vi "Alarm Logical Channel.vi"(8 "error in (no error)":errorcluster, 9 "12 Logicals inputs state":T1[](array[typedef]) items=["Off", "On", "Ignore"], 10 "Alarm":u16(ring) items=["A", "B", "C", "D"], 11 "VISA resource name":refnum<visa-resource-name>) -> (0 "error out":errorcluster, 3 "VISA resource name out":refnum<visa-resource-name>)   [LabVIEW 2017, in "Sefram DAS220.lvlib"]
doc: "Alarm trigs on logical channels trigger."
uses:
  <instrlib>/Sefram DAS220/Sefram DAS220.lvlib
  <instrlib>/Sefram DAS220/Public/Configure/Triggers-Alarms/Low-level/Trigger Types/Logical TriState.ctl
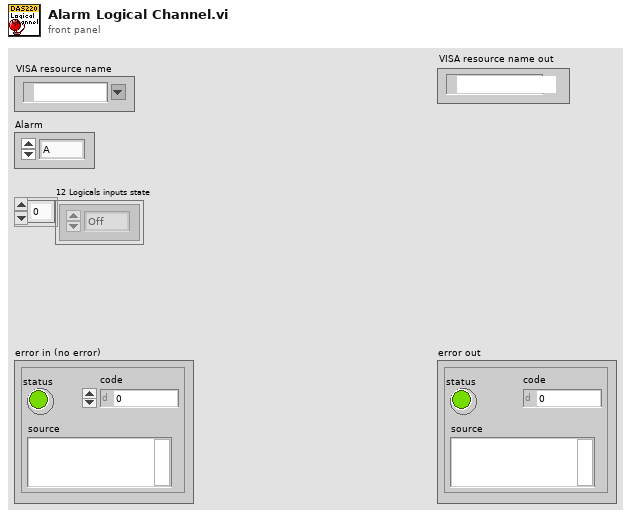
[diagram p1: front panel]
types:
  T1 = typedef "Sefram DAS220.lvlib/Logical TriState.ctl" = u16
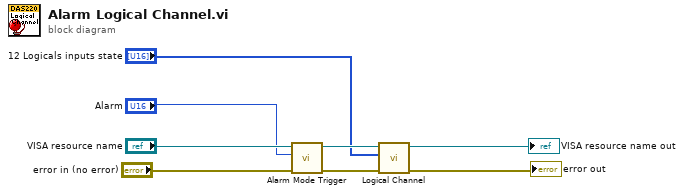
[diagram p0: block diagram]
diagram:
  n1 = call <instrlib>:"Alarm Mode Trigger.vi"("error in (no error)"="error in (no error)", "Alarm"="Alarm", "VISA resource name"="VISA resource name") -> ("error out"=w5:errorcluster, "VISA resource name out"=w6:refnum<visa-resource-name>)  [unwired: 7 in]
  n2 = call <instrlib>:"Logical Channel.vi"("error in (no error)"=w5, "12 Logicals inputs state"="12 Logicals inputs state", "VISA resource name"=w6) -> ("error out"=→"error out":errorcluster, "VISA resource name out"=→"VISA resource name out":refnum<visa-resource-name>)  [unwired: 7 in]
